vi "ExpVar Init.vi"(8 "error in":errorcluster) -> (0 "error out":errorcluster, 3 "NewExpVar.lvclass":refnum<class "ExpVar.lvclass">)   [LabVIEW 2018, in "ExpVar.lvclass"]
uses:
  ExpVar.lvclass
  ExpVar.lvclass/ExpVar.ctl
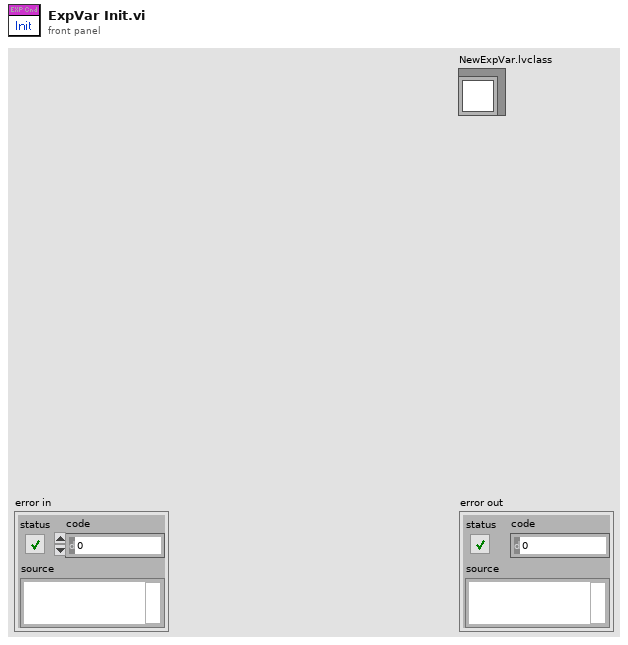
[diagram p1: front panel]
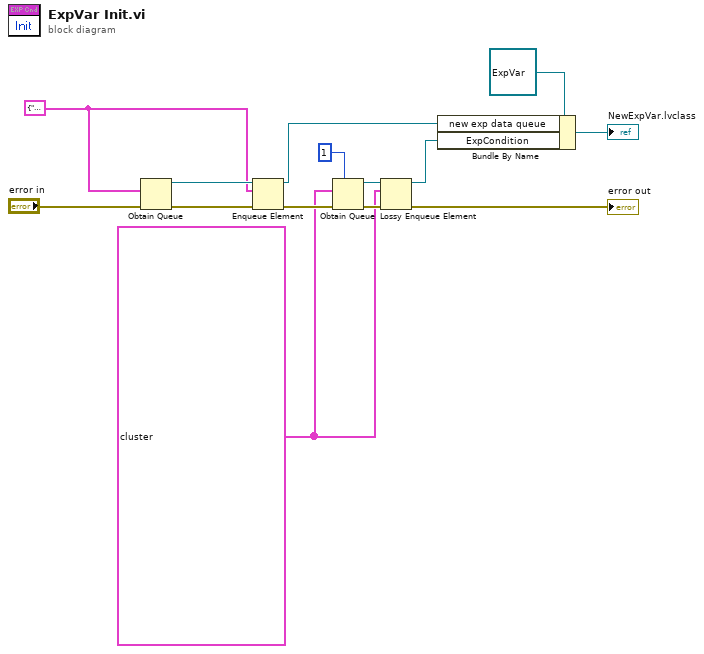
[diagram p0: block diagram]
diagram:
  w2 = cluster{"Label":string, "Value":variant}[] [{"Label"="Laser", "Value"=variant}, {"Label"="Pressure", "Value"=variant}, {"Label"="TMP", "Value"=variant}, {"Label"="Script", "Value"=variant}, {"Label"="Signal Remarks", "Value"=variant}, {"Label"="ExtAO", "Value"=variant}, {"Label"="ExtDO", "Value"=variant}, {"Label"="ExtDI", "Value"=variant}, {"Label"="DAQ", "Value"=variant}] ("ExpCondi")
  w1 = cluster{"Label":string, "Value":variant} {"Label"="", "Value"=variant}
  n1 = Obtain Queue(element data type=w1, error in (no error)="error in") -> (queue out=w12:refnum<queue>, error out=w9:errorcluster)  [unwired: 3 in, 1 out]
  n2 = Enqueue Element(queue=w12, element=w1, error in (no error)=w9) -> (queue out=w10:refnum<queue>, error out=w8:errorcluster)  [unwired: 1 in, 1 out]
  n3 = Obtain Queue(max queue size (-1, unlimited)=1, element data type=w2, error in (no error)=w8) -> (queue out=w7:refnum<queue>, error out=w4:errorcluster)  [unwired: 2 in, 1 out]
  n4 = Lossy Enqueue Element(queue=w7, element=w2, error in (no error)=w4) -> (queue out=w5:refnum<queue>, error out=→"error out":errorcluster)  [unwired: 2 out]
  n5 = Bundle By Name(cluster=refnum<class "ExpVar.lvclass"> refnum ("NewExpVar.lvclass 2"), "new exp data queue"=w10, "ExpCondition"=w5) -> (→"NewExpVar.lvclass":refnum<class "ExpVar.lvclass">)
